vi "EnFlo_Error_Handler.vi"(3 "error in (no error)":errorcluster, 4 "Error Type":string, 5 "Dialog Box (F)":bool) -> (0 "Continue":bool, 2 "Email Message":string)   [LabVIEW 2022 SP3]
uses:
  <vilib>/Utility/error.llb/DialogType.ctl
  Globals/Meas_global.vi
  Globals/Trav_pos_global.vi
  Globals/Preference_global.vi
  Email_transfer_global.vi
panel:
  out "error out":errorcluster
  out "Hours Running":dbl format="%.2f"
  out "Error Information":string
  out "Log Files":path[](array[path])
  out "nOccurences":i32
  out "Error Analysis":string
  out "Error Types":string[](array[string])
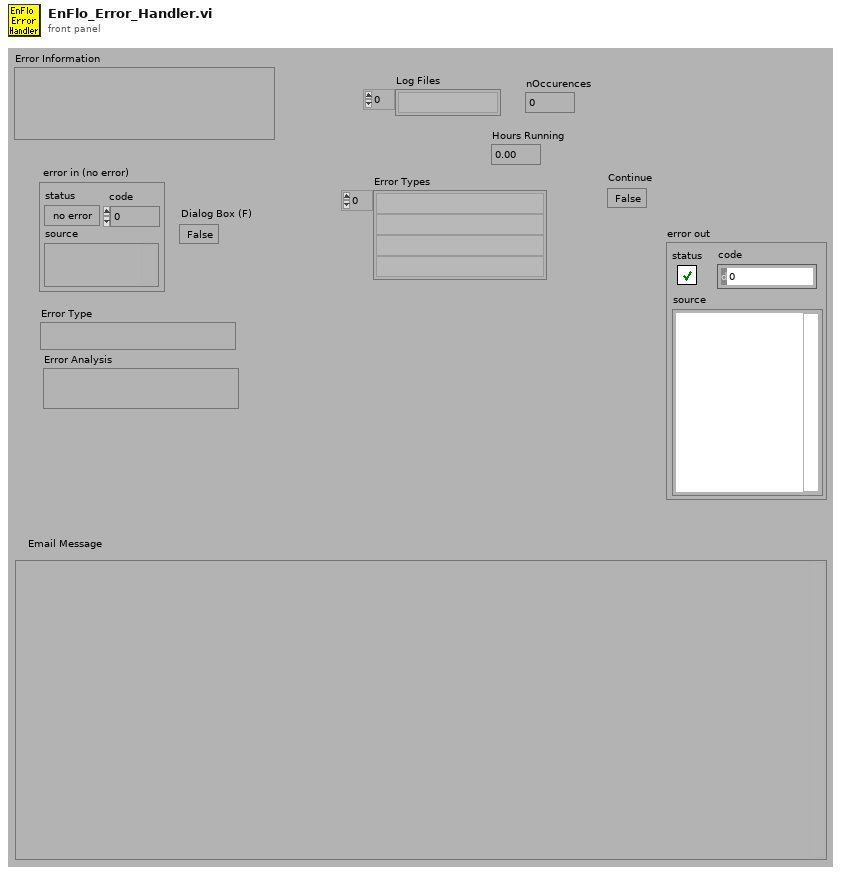
[diagram p1: front panel]
types:
  T1 = typedef "DialogType.ctl" = u16
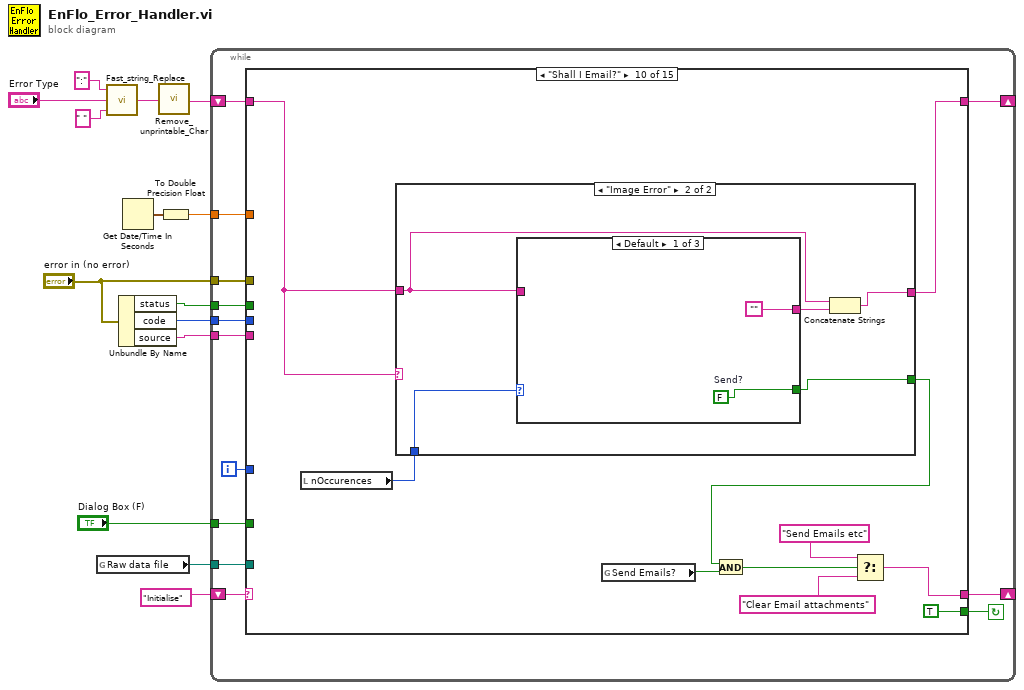
[diagram p0: block diagram]
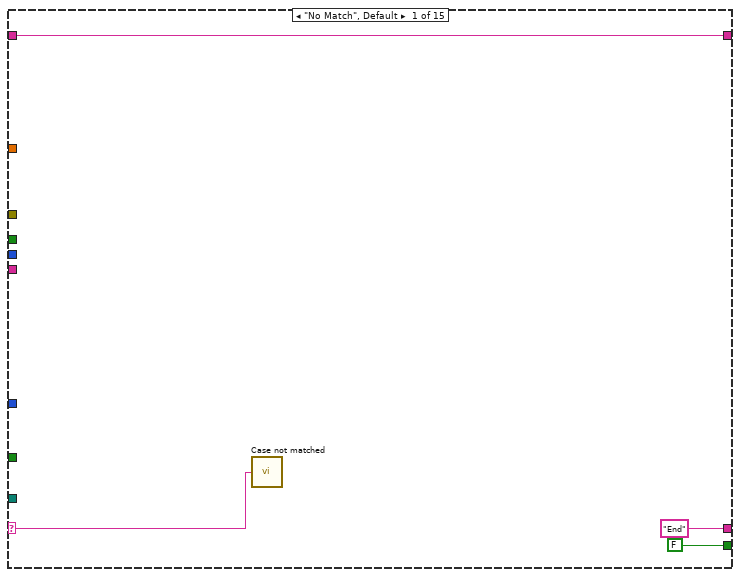
[diagram p2: hidden frame]
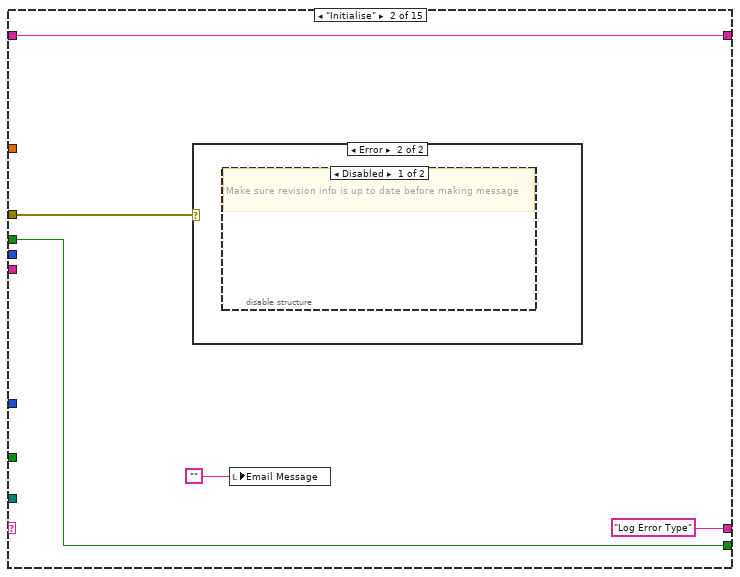
[diagram p3: hidden frame]
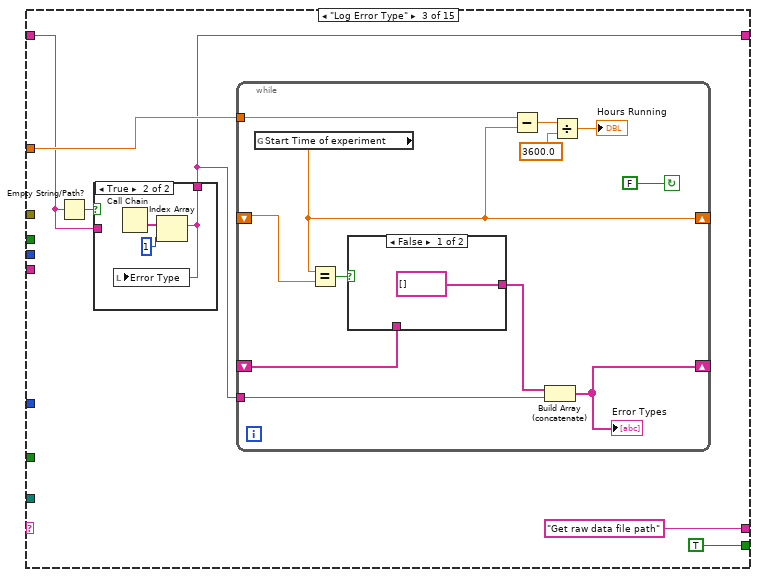
[diagram p6: hidden frame]
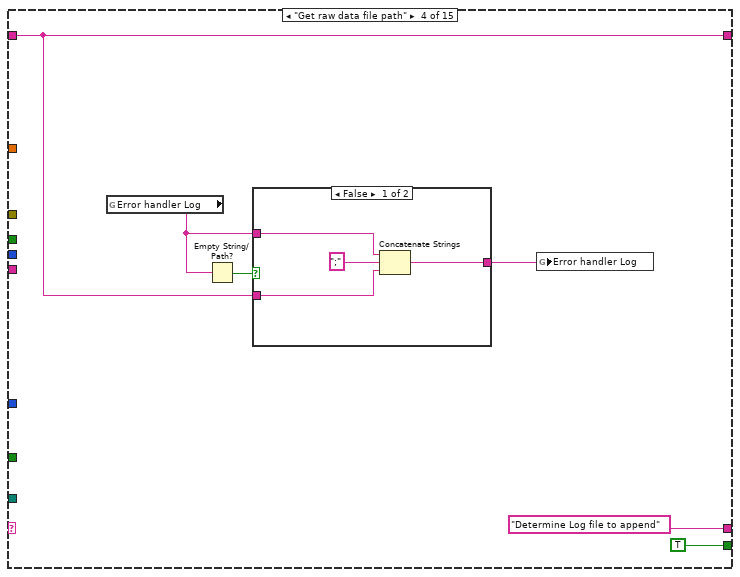
[diagram p9: hidden frame]
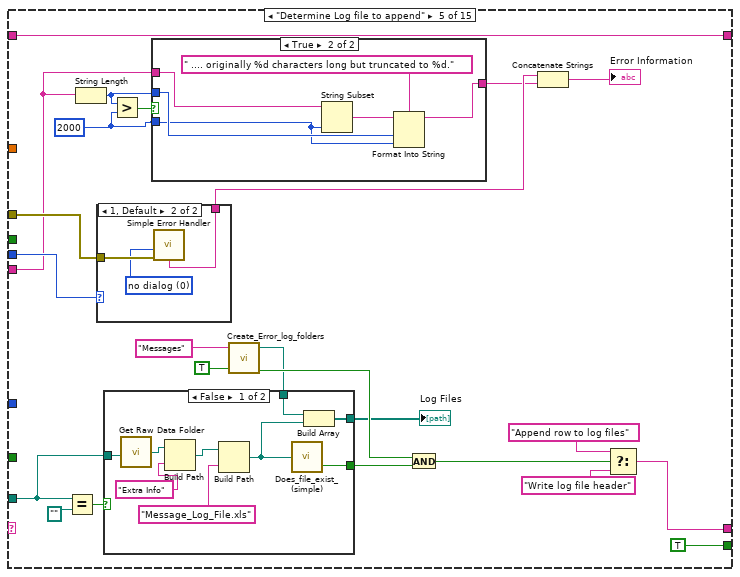
[diagram p11: hidden frame]
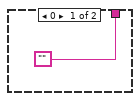
[diagram p13: hidden frame]
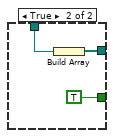
[diagram p14: hidden frame]
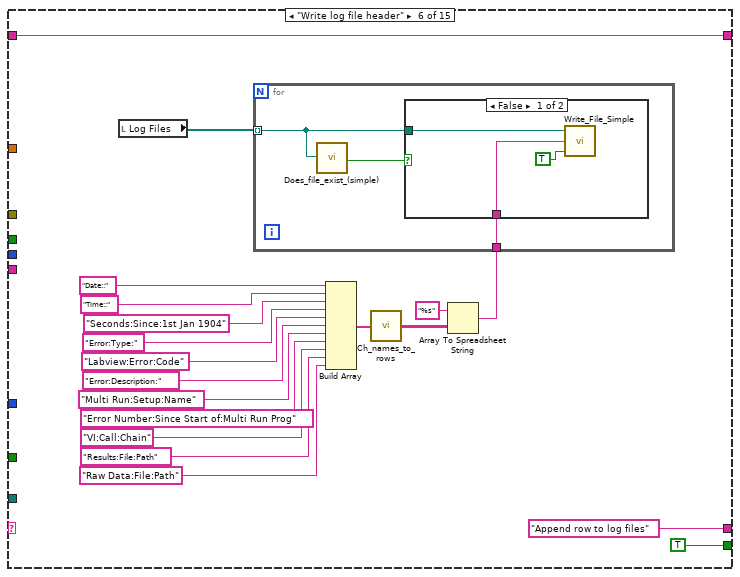
[diagram p15: hidden frame]
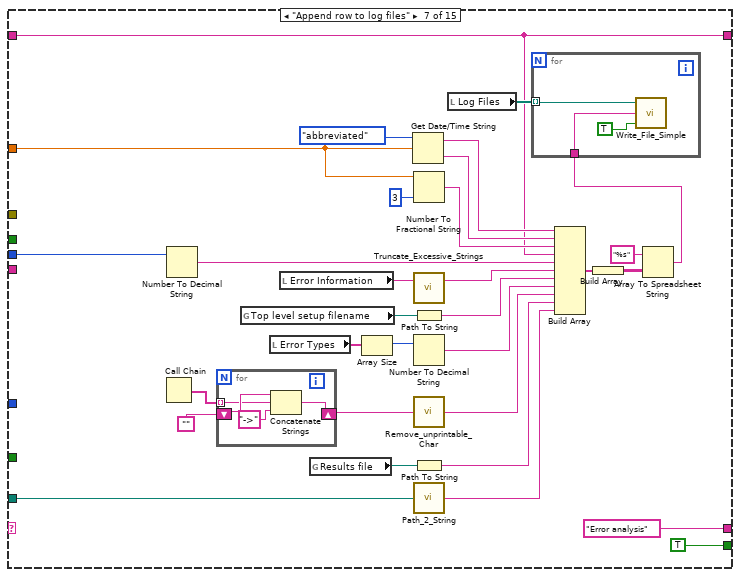
[diagram p17: hidden frame]
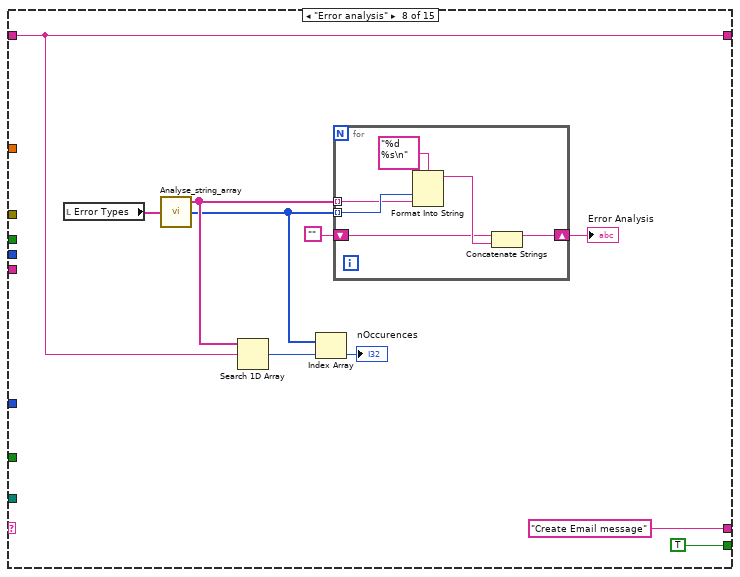
[diagram p18: hidden frame]
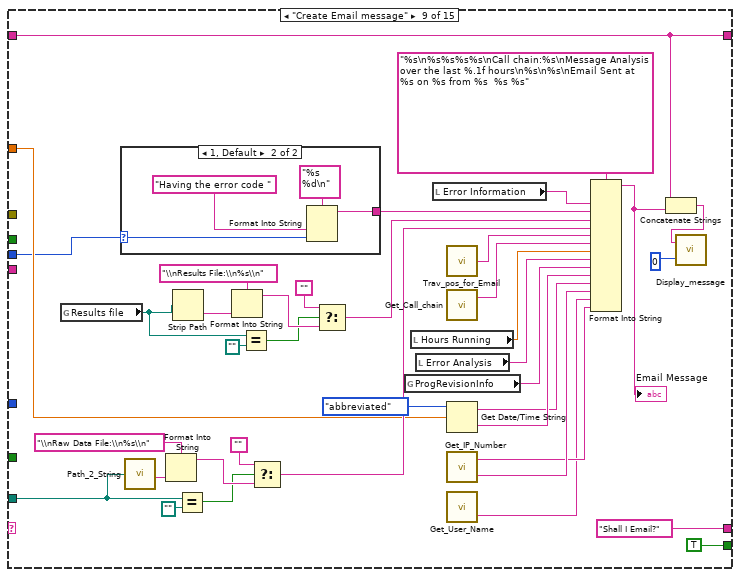
[diagram p19: hidden frame]
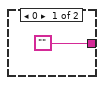
[diagram p20: hidden frame]
diagram:
  n1 = global read "Meas_global.vi" "Raw data file"() -> (w6:path)
  n2 = call "Fast_string_Replace.vi"("Replace match with:"=" ", "Input String"="Error Type", "matchThis"=":" ("regular expression")) -> ("Output String"=w2:string)  [unwired: 1 in, 1 out]
  n3 = Unbundle By Name("error in (no error)") -> ("status"=w13:bool, "code"=w12:i32, "source"=w11:string)
  n4 = Get Date/Time In Seconds() -> (seconds since 1Jan1904=w10:timestamp)
  n5 = call "Remove_unprintable_Char.vi"("Input String"=w2) -> ("Output String"=w1:string)
  n6 = To Double Precision Float(number=w10) -> (double precision float=w14:dbl)
  n7 = while {
    tunnel: w11 -> [w21]
    tunnel: w12 -> [w23]
    tunnel: w13 -> [w24]
    tunnel: w14 -> [w25]
    shift-left: "Initialise" -> [w20]
    shift-right: [w26] -> _
    shift-right: [w18] -> _
    shift-left: w1 -> [w19]
    tunnel: "Dialog Box (F)" -> [w17]
    tunnel: "error in (no error)" -> [w16]
    tunnel: w6 -> [w15]
    i -> [w22]
    stop <- w27 continue-if-true
    n8 = case shown="\"Shall I Email?\"" w20 {
      selector: w20 -> [w28 _ _ _ _ _ _ _ _ _ _ _ _ _ _]
      tunnel: [FALSE ("Abort") w36 TRUE ("status") TRUE ("status") TRUE ("status") TRUE TRUE TRUE ("status") TRUE ("Abort") TRUE ("Abort") TRUE ("Abort") TRUE ("Abort") w318 w326 FALSE ("Abort")] -> w27
      tunnel: ["End" ("f") "Log Error Type" "Get raw data file path" ("f") "Determine Log file to append" ("f") w93 "Append row to log files" ("f") "Error analysis" ("f") "Create Email message" ("f") "Shall I Email?" w250 "Clear Email attachments" "Is ADAM scan table running?" ("f") "Show timed error dialog" "Stop" "End"] -> w26
      tunnel: w25 -> [_ _ w40 _ _ _ w151 _ w216 _ _ _ _ _ _]
      tunnel: w24 -> [_ w36 _ _ _ _ _ _ _ _ _ _ _ _ _]
      tunnel: w23 -> [_ _ _ _ w79 _ w169 _ w198 _ _ _ _ _ _]
      tunnel: w22 -> [_ _ _ _ _ _ _ _ _ _ _ _ _ _ _]
      tunnel: w21 -> [_ _ _ _ w75 _ _ _ _ _ _ _ _ _ _]
      tunnel: w19 -> [w29 w33 w38 w64 w83 w119 w148 w183 w203 w241 w285 w315 w319 w324 w330]
      tunnel: [w29 w33 w37 w64 w83 w119 w148 w183 w203 w242 w285 w315 w319 w324 w330] -> w18
      tunnel: w17 -> [_ _ _ _ _ _ _ _ _ _ _ _ w317 _ _]
      tunnel: w16 -> [_ w32 _ _ w81 _ _ _ _ _ _ _ _ _ _]
      tunnel: w15 -> [_ _ _ _ w78 _ w146 _ w208 _ _ _ _ _ _]
      frame "No Match", Default {
        n9 = call "Case not matched.vi"("Case Name not Matched"=w28) -> ()
      }
      frame "Initialise" {
        n10 = case shown="Error" w32 {
          frame No Error {
          }
          frame Error {
            n11 = disable-structure shown="Disabled" {
              frame Disabled {
                # "Make sure revision info is up to date before making message"
              }
              frame Enabled {
              }
            }
          }
        }
        n12 = local write "Email Message"("") -> ()
      }
      frame "Log Error Type" {
        n13 = Empty String/Path?(string/path=w38) -> (empty?=w41:bool)
        n14 = case shown="True" w41 {
          tunnel: w38 -> [w57 _]
          tunnel: [w57 w58] -> w37
          frame False {
          }
          frame True {
            n15 = Call Chain() -> (call chain=w60:string[])
            n16 = Index Array(array=w60, index=1 ("Index")) -> (element=w58:string)
            n17 = local write "Error Type"(w58) -> ()
          }
        }
        n18 = while {
          tunnel: w40 -> [w45]
          shift-left: _ -> [w52]
          shift-right: [w51] -> _
          shift-left: _ -> [w50]
          shift-right: [w48] -> _
          tunnel: w37 -> [w53]
          stop <- FALSE continue-if-true
          n19 = global read "Meas_global.vi" "Start Time of experiment"() -> (w48:dbl)
          n20 = Equal?(x=w48, y=w50) -> (x = y?=w49:bool)
          n21 = case shown="False" w49 {
            tunnel: [string[] [] w56] -> w54
            tunnel: w52 -> [_ w56]
            frame False {
            }
            frame True {
            }
          }
          n22 = Subtract(x=w45, y=w48) -> (x-y=w47:dbl)
          n23 = Build Array (concatenate)(w54, w53) -> (w51:string[])
          "Error Types" <- w51
          n24 = Divide(x=w47, y=3600.0) -> (x/y=→"Hours Running":dbl)
        }
      }
      frame "Get raw data file path" {
        n25 = global read "Meas_global.vi" "Error handler Log"() -> (w62:string)
        n26 = Empty String/Path?(string/path=w62) -> (empty?=w61:bool)
        n27 = case shown="False" w61 {
          tunnel: w64 -> [w70 w71]
          tunnel: [w68 w71] -> w63
          tunnel: w62 -> [w67 _]
          frame False {
            n28 = Concatenate Strings(w67, ";" ("string"), w70) -> (w68:string)
          }
          frame True {
          }
        }
        n29 = global write "Meas_global.vi" "Error handler Log"(w63) -> ()
      }
      frame "Determine Log file to append" {
        w73 = 2000 ("length (rest)")
        n30 = Equal?(x=w78, y=path "") -> (x = y?=w91:bool)
        n31 = String Length(string=w75) -> (length=w72:i32)
        n32 = case shown="1, Default" w79 {
          tunnel: w81 -> [_ w106]
          tunnel: ["" w104] -> w80
          frame 0 {
          }
          frame 1, Default {
            w105 = T1 0 items=["no dialog", "OK message", "continue or stop message", "OK message + warnings", "continue/stop + warnings"] ("type of dialog (OK msg:1)")
            n33 = call <vilib>:"Simple Error Handler.vi"("type of dialog (OK msg:1)"=w105, "error in (no error)"=w106) -> ("message"=w104:string)  [unwired: 7 out]
          }
        }
        n34 = Greater?(x=w72, y=w73) -> (0:w74:bool)
        n35 = case shown="True" w74 {
          tunnel: [w96 w97] -> w76
          tunnel: w75 -> [w96 w102]
          tunnel: w73 -> [_ w100]
          tunnel: w72 -> [_ w101]
          frame False {
          }
          frame True {
            n36 = String Subset(string=w102, length (rest)=w100) -> (substring=w98:string)  [unwired: 1 in]
            n37 = Format Into String(format string=" .... originally %d characters long but truncated to %d.", initial string=w98, w101, w100) -> (resulting string=w97:string)  [unwired: 1 in, 1 out]
          }
        }
        n38 = call "Create_Error_log_folders.vi"("Log Filename"="Messages" ("Input Element"), "Per Day Log File?"=TRUE) -> ("Local Log File"=w87:path, "exists?"=w89:bool)  [unwired: 4 in]
        n39 = case shown="False" w91 {
          tunnel: w78 -> [w108 _]
          tunnel: [w114 TRUE ("exists?")] -> w90
          tunnel: w87 -> [w113 w117]
          tunnel: [w111 w116] -> w86
          frame False {
            n40 = call "Get Raw Data Folder.vi"("Raw data file"=w108) -> ("Main Raw Data Folder"=w107:path)
            n41 = Build Path(base path=w107, name or relative path="Extra Info") -> (appended path=w109:path)
            n42 = Build Path(base path=w109, name or relative path="Message_Log_File.xls") -> (appended path=w112:path)
            n43 = call "Does_file_exist_(simple).vi"("Pathname"=w112) -> ("exists?"=w114:bool)
            n44 = Build Array(w113, w112) -> (w111:path[])
          }
          frame True {
            n45 = Build Array(w117) -> (w116:path[])
          }
        }
        "Log Files" <- w86
        n46 = And(x=w89, y=w90) -> (x .and. y?=w88:bool)
        n47 = Concatenate Strings(w80, w76) -> (→"Error Information":string)
        n48 = Select(t="Append row to log files", s=w88, f="Write log file header") -> (s? t:f=w93:string)
      }
      frame "Write log file header" {
        n49 = local read "Log Files"() -> (w123:path[])
        n50 = Build Array("Date::", "Time::", "Seconds:Since:1st Jan 1904", "Error:Type:", "Labview:Error:Code", "Error:Description:", "Multi Run:Setup:Name", "Error Number:Since Start of:Multi Run Prog", "VI:Call:Chain", "Results:File:Path", "Raw Data:File:Path") -> (w122:string[])
        n51 = call "Ch_names_to_rows.vi"("Channel Names"=w122) -> ("3 Row names"=w121:string[][])
        n52 = Array To Spreadsheet String(array=w121, 3:"%s" ("format string")) -> (spreadsheet string=w127:string)  [unwired: 1 out]
        n53 = for {
          tunnel: w127 -> [w140]
          tunnel: w123 -> [w138] mode=indexing
          n54 = call "Does_file_exist_(simple).vi"("Pathname"=w138) -> ("exists?"=w139:bool)
          n55 = case shown="False" w139 {
            tunnel: w140 -> [w142 _]
            tunnel: w138 -> [w141 _]
            frame False {
              n56 = call "Write_File_Simple.vi"("append to file? (new file:F)"=TRUE, "character string"=w142, "file path"=w141) -> ()  [unwired: 2 out]
            }
            frame True {
            }
          }
        }
      }
      frame "Append row to log files" {
        n57 = Call Chain() -> (call chain=w160:string[])
        n58 = Number To Decimal String(number=w169) -> (decimal integer string=w168:string)  [unwired: 1 out]
        n59 = for {
          shift-right: [w178] -> w159
          shift-left: "" -> [w181]
          tunnel: w160 -> [w180] mode=indexing
          n60 = Concatenate Strings(w181, w180, "->" ("Substring")) -> (w178:string)
        }
        n61 = global read "Trav_pos_global.vi" "Top level setup filename"() -> (w171:path)
        n62 = local read "Error Types"() -> (w165:string[])
        n63 = local read "Error Information"() -> (w145:string)
        n64 = global read "Meas_global.vi" "Results file"() -> (w155:path)
        n65 = Array Size(array=w165) -> (size(s)=w170:i32)
        n66 = Get Date/Time String(date format (0)=enum16{"short", "long", "abbreviated"}."abbreviated", seconds (now)=w151) -> (date string=w173:string, time string=w172:string)  [unwired: 1 out]
        n67 = Number To Fractional String(number=w151, precision (6)=i16 3) -> (F-format string=w150:string)  [unwired: 2 out]
        n68 = call "Truncate_Excessive_Strings.vi"("String"=w145) -> ("Truncated String"=w144:string)  [unwired: 2 in]
        n69 = Path To String(path=w171) -> (string=w167:string)
        n70 = Number To Decimal String(number=w170) -> (decimal integer string=w166:string)  [unwired: 1 out]
        n71 = call "Remove_unprintable_Char.vi"("Input String"=w159) -> ("Output String"=w161:string)
        n72 = Path To String(path=w155) -> (string=w154:string)
        n73 = call "Path_2_String.vi"("Real Path"=w146) -> ("Path String"=w147:string)
        n74 = local read "Log Files"() -> (w153:path[])
        n75 = Build Array(w173, w172, w150, w148, w168, w144, w167, w166, w161, w154, w147) -> (w156:string[])
        n76 = Build Array(w156) -> (w164:string[][])
        n77 = Array To Spreadsheet String(array=w164, 3:"%s" ("format string")) -> (spreadsheet string=w162:string)  [unwired: 1 out]
        n78 = for {
          tunnel: w162 -> [w176]
          tunnel: w153 -> [w175] mode=indexing
          n79 = call "Write_File_Simple.vi"("append to file? (new file:F)"=TRUE, "character string"=w176, "file path"=w175) -> ()  [unwired: 2 out]
        }
      }
      frame "Error analysis" {
        n80 = local read "Error Types"() -> (w186:string[])
        n81 = call "Analyse_string_array.vi"("String array"=w186) -> ("Unique strings"=w190:string[], "Frequency"=w189:i32[])  [unwired: 1 out]
        n82 = Search 1D Array(1D array=w190, element=w183) -> (index of element=w191:i32)  [unwired: 1 out]
        n83 = Index Array(array=w189, index=w191) -> (element=→"nOccurences":i32)
        n84 = for {
          tunnel: w190 -> [w195] mode=indexing
          tunnel: w189 -> [w196] mode=indexing
          shift-right: [w192] -> w187
          shift-left: "" -> [w193]
          n85 = Format Into String(format string="%d %s\n" ("Format String"), w196, w195) -> (resulting string=w194:string)  [unwired: 2 in, 1 out]
          n86 = Concatenate Strings(w193, w194) -> (w192:string)
        }
        "Error Analysis" <- w187
      }
      frame "Create Email message" {
        n87 = global read "Meas_global.vi" "Results file"() -> (w207:path)
        n88 = case shown="1, Default" w198 {
          selector: w198 -> [_ w237]
          tunnel: ["" w238] -> w235
          frame 0 {
          }
          frame 1, Default {
            n89 = Format Into String(format string="%s %d\n" ("Format String"), "Having the error code ", w237) -> (resulting string=w238:string)  [unwired: 2 in, 1 out]
          }
        }
        n90 = call "Path_2_String.vi"("Real Path"=w208) -> ("Path String"=w210:string)
        n91 = Format Into String(format string="\\nRaw Data File:\\n%s\\n" ("Format String"), w210) -> (resulting string=w225:string)  [unwired: 2 in, 1 out]
        n92 = Strip Path(path=w207) -> (name=w206:string)  [unwired: 1 out]
        n93 = Equal?(x=w208, y=path "") -> (x = y?=w222:bool)
        n94 = Format Into String(format string="\\nResults File:\\n%s\\n" ("Format String"), w206) -> (resulting string=w227:string)  [unwired: 2 in, 1 out]
        n95 = Equal?(x=w207, y=path "") -> (x = y?=w221:bool)
        n96 = Select(t="", s=w222, f=w225) -> (s? t:f=w229:string)
        n97 = Select(t="", s=w221, f=w227) -> (s? t:f=w230:string)
        n98 = global read "Meas_global.vi" "ProgRevisionInfo"() -> (w204:string)
        n99 = local read "Hours Running"() -> (w218:dbl)
        n100 = local read "Error Analysis"() -> (w217:string)
        n101 = local read "Error Information"() -> (w220:string)
        n102 = call "Trav_pos_for_Email.vi"() -> ("String"=w219:string)
        n103 = call "Get_Call_chain.vi"() -> ("Output String"=w205:string)  [unwired: 1 in, 1 out]
        n104 = Get Date/Time String(date format (0)=enum16{"short", "long", "abbreviated"}."abbreviated", seconds (now)=w216) -> (date string=w213:string, time string=w214:string)  [unwired: 1 out]
        n105 = call "Get_IP_Number.vi"() -> ("bestAvailableName"=w209:string, "IP Number"=w200:string)
        n106 = call "Get_User_Name.vi"() -> ("User Name"=w199:string)  [unwired: 1 in]
        n107 = Format Into String(format string="%s\n%s%s%s%s\nCall chain:%s\nMessage Analysis over the last %.1f hours\n%s\n%s\nEmail Sent at %s on %s from %s  %s %s" ("Format String"), w220, w235, w230, w229, w219, w205, w218, w217, w204, w214, w213, w209, w199, w200) -> (resulting string=w202:string)  [unwired: 2 in, 1 out]
        "Email Message" <- w202
        n108 = Concatenate Strings(w203, w202) -> (w201:string)
        n109 = call "Display_message.vi"("Time to display message"=u32 0, "Message"=w201) -> ()  [unwired: 2 out]
      }
      frame "Shall I Email?" {
        n110 = local read "nOccurences"() -> (w246:i32)
        n111 = case shown="\"Image Error\"" w241 {
          tunnel: [w253 w270] -> w244
          tunnel: w246 -> [w255 w272]
          tunnel: [w251 w268] -> w242
          tunnel: w241 -> [w254 w271]
          frame Default {
            n112 = case shown="200" w255 {
              selector: w255 -> [_ w260 _ w265]
              tunnel: [w257 w261 w263 w267] -> w253
              tunnel: w254 -> [_ _ _ _]
              tunnel: ["" w258 "" w266] -> w252
              frame Default {
                w257 = FALSE  # Send?
              }
              frame 10, 50, 100 {
                w261 = TRUE  # Send Message
                n113 = Format Into String(format string="%dth REPEATED MESSAGE", w260) -> (resulting string=w258:string)  [unwired: 2 in, 1 out]
              }
              frame 1 {
                w263 = TRUE  # Send Message
              }
              frame 200 {
                w267 = TRUE  # Send Message
                n114 = Format Into String(format string="%dth REPEATED MESSAGE FINAL WARNING!!", w265) -> (resulting string=w266:string)  [unwired: 2 in, 1 out]
              }
            }
            n115 = Concatenate Strings(w254, w252) -> (w251:string)
          }
          frame "Image Error" {
            n116 = case shown="Default" w272 {
              selector: w272 -> [_ w277 w280]
              tunnel: [w274 w278 w282] -> w270
              tunnel: w271 -> [_ _ _]
              tunnel: ["" w275 w281] -> w269
              frame Default {
                w274 = FALSE  # Send?
              }
              frame 6, 60 {
                w278 = TRUE  # Send Message
                n117 = Format Into String(format string="%dth Repeated Message", w277) -> (resulting string=w275:string)  [unwired: 2 in, 1 out]
              }
              frame 600 {
                w282 = TRUE  # Send Message
                n118 = Format Into String(format string="%dth Repeated Message, final warning.", w280) -> (resulting string=w281:string)  [unwired: 2 in, 1 out]
              }
            }
            n119 = Concatenate Strings(w271, w269) -> (w268:string)
          }
        }
        n120 = global read "Preference_global.vi" "Send Emails?"() -> (w245:bool)
        n121 = And(x=w244, y=w245) -> (x .and. y?=w243:bool)
        n122 = Select(t="Send Emails etc", s=w243, f="Clear Email attachments") -> (s? t:f=w250:string)
      }
      frame "Send Emails etc" {
        n123 = global read "Preference_global.vi" "LabVIEW Administrators"() -> (w283:string[])
        n124 = stacked-sequence {
          tunnel: w285 -> [_ w291 _ _]
          tunnel: w283 -> [w288 _ w305 _]
          frame #0 {
            n125 = global read "Meas_global.vi" "People to Email"() -> (w287:string[])
            n126 = global read "Email_transfer_global.vi" "recipients"() -> (w289:string[])
            n127 = Build Array (concatenate)(w289, w288, w287) -> (w290:string[])
            n128 = global write "Email_transfer_global.vi" "recipients"(w290) -> ()
          }
          frame #1 {
            n129 = global write "Email_transfer_global.vi" "subject ([No Subject])"(w291) -> ()
          }
          frame #2 {
            n130 = local read "Email Message"() -> (w292:string)
            n131 = Concatenate Strings(w292, "\nThis email has been generated  automatically by LabVIEW. If you need help with understanding the email, or want to be removed from the mailing list please contact:\n") -> (w303:string)
            n132 = Concatenate Strings(" or ", "\r\n") -> (w299:string)
            n133 = for {
              shift-right: [w307] -> w302
              shift-left: w303 -> [w309]
              tunnel: w305 -> [w308] mode=indexing
              tunnel: w299 -> [w306]
              n134 = Concatenate Strings(w309, w308, w306) -> (w307:string)
            }
            n135 = String Length(string=w299) -> (length=w297:i32)
            n136 = String Length(string=w302) -> (length=w298:i32)
            n137 = Subtract(x=w298, y=w297) -> (x-y=w296:i32)
            n138 = String Subset(string=w302, length (rest)=w296) -> (substring=w295:string)  [unwired: 1 out]
            n139 = Concatenate Strings(w295, "\r\n") -> (w293:string)
            n140 = global write "Email_transfer_global.vi" "message"(w293) -> ()
          }
          frame #3 {
            n141 = call "Launch_Async_Email.vi"() -> ("error out"=→"error out":errorcluster)  [unwired: 2 out]
          }
        }
      }
      frame "Clear Email attachments" {
        n142 = global write "Email_transfer_global.vi" "attachments"(path[] [] ("attachments")) -> ()
        n143 = global write "Email_transfer_global.vi" "recipients"(string[] [] ("recipients")) -> ()
      }
      frame "Is ADAM scan table running?" {
        n144 = Open VI Reference(vi path="ADAM_scan_table.vi") -> (vi reference=w322:refnum<vi>, error out=w316:errorcluster)  [unwired: 1 in, 4 out]
        n145 = case shown="No Error" w316 {
          tunnel: w322 -> [w323 _]
          frame No Error {
            n146 = Close Reference(reference=w323) -> ()  [unwired: 1 in, 1 out]
          }
          frame Error {
          }
        }
        n147 = Compound Arithmetic op=AND(w316, w317) -> (w318:bool)
      }
      frame "Show timed error dialog" {
        n148 = local read "Email Message"() -> (w328:string)
        n149 = call "Timed_Error_dialog.vi"("Message"=w328, "Seconds to wait"=60.0) -> ("Ignore"=→"Continue":bool, "Abort"=w326:bool)
      }
      frame "Stop" {
        n150 = stacked-sequence {
          seq-local: [_ w340 _ _] -> [_ _ w354 _]
          frame #0 {
            n151 = call "Program_Active_Aborting.vi"() -> ()  [unwired: 6 out]
          }
          frame #1 {
            n152 = Build Array("Edit_BSA_setup.vi", "Measurement_input_panel.vi", "Input_Value_Dialog.vi", "Input_String_Dialog.vi", "Calibration_user_input.vi", "Input_Traverse_position.vi", "User_Metadata.vi", "Preference_Panel.vi", "Traverse_Space.vi", "Enter_Temp_Press.vi", "EnFlo_Tunnel_Setup.vi", "Gas_Setup.vi", "Correlation_Display.vi", "Serial_Setup.vi", "Port_Names.vi", "Select_Strings.vi", "Edit_Template_File.vi", "Select_a_Channel.vi", "Output_file_Panel.vi", "Enter_LDA_Setup.vi") -> (w340:string[])
          }
          frame #2 {
            n153 = for {
              tunnel: w354 -> [w355] mode=indexing
              n154 = Open VI Reference(vi path=w355) -> (vi reference=w359:refnum<vi>, error out=w358:errorcluster)  [unwired: 1 in, 4 out]
              n155 = property class="VI"(reference=w359, error in=w358, "Front Panel Window:Open"=FALSE) -> (reference out=w357:refnum<vi>)  [unwired: 1 out]
              n156 = Close Reference(reference=w357) -> ()  [unwired: 1 in, 1 out]
            }
          }
          frame #3 {
            n157 = Stop(stop? (T)=TRUE) -> ()
          }
        }
      }
    }
  }
